vi "Read SC2250 TX Resource Name.vi"(8 "error in (no error)":errorcluster, 11 "SG SC2250 Path in":refnum<class "SG SC2250 Path.lvclass">) -> (0 "error out":errorcluster, 2 "SC2250 TX Resource Name":string, 3 "SG SC2250 Path out":refnum<class "SG SC2250 Path.lvclass">)   [LabVIEW 2023, in "RFFixtureCharact.RFPM.lvlib" / "SG SC2250 Path.lvclass"]
uses:
  SG SC2250 Path.lvclass
  SG SC2250 Path.lvclass/SG SC2250 Path.ctl
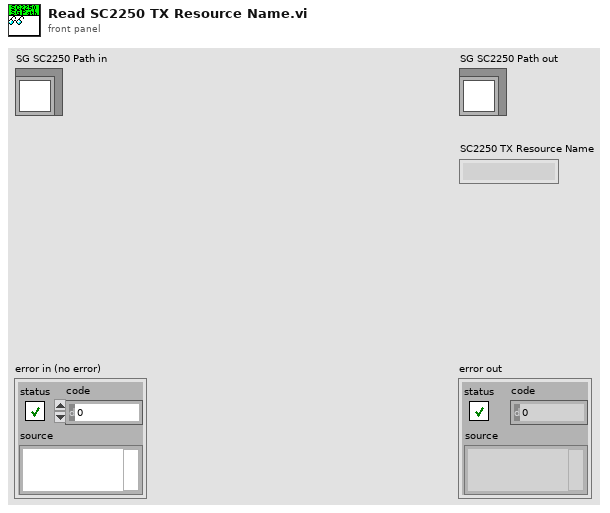
[diagram p1: front panel]
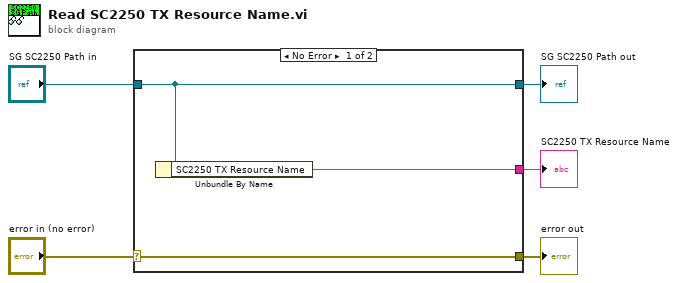
[diagram p0: block diagram]
diagram:
  n1 = case shown="No Error" "error in (no error)" {
    selector: "error in (no error)" -> [w8 w9]
    tunnel: [w8 w9] -> w4
    tunnel: [w7 w10] -> w2
    tunnel: "SG SC2250 Path in" -> [w7 w10]
    tunnel: [w6 _] -> w1
    frame No Error {
      n2 = Unbundle By Name(w7) -> ("SC2250 TX Resource Name"=w6:string)
    }
    frame Error {
    }
  }
  "error out" <- w4
  "SG SC2250 Path out" <- w2
  "SC2250 TX Resource Name" <- w1
